vi "Min & Max Data display in graph.vi"() -> ()   [LabVIEW 2015]
panel:
  out "Waveform Graph":i32[](graph)
  # "Min & Max Data display in graph"
  # "Pardeep Kumar"
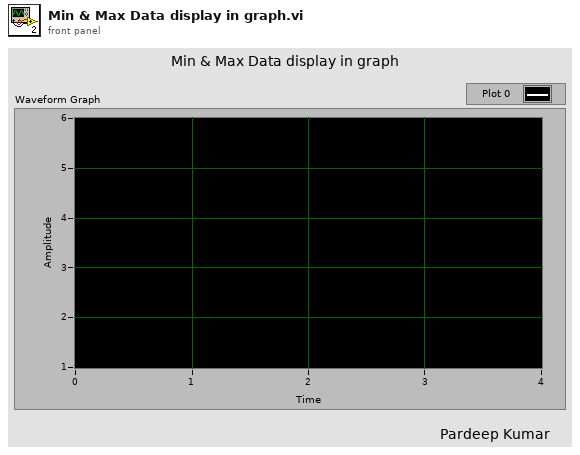
[diagram p1: front panel]
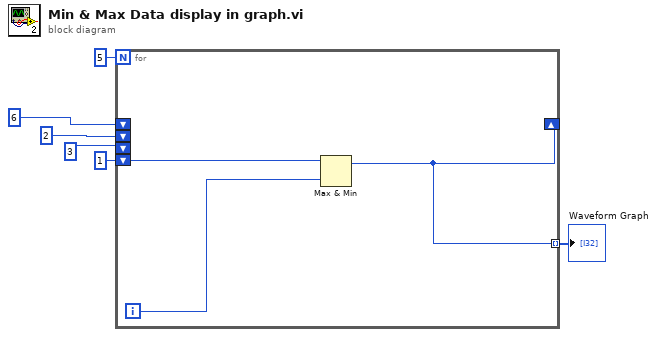
[diagram p0: block diagram]
diagram:
  n1 = for {
    N: 5 -> [_]
    shift-right: [w7] -> _
    shift-left: 1 -> [w8]
    shift-left: 3 -> [_]
    shift-left: 2 -> [_]
    shift-left: 6 -> [_]
    tunnel: [w7] -> w1 mode=indexing
    i -> [w9]
    n2 = Max & Min(x=w8, y=w9) -> (max(x,y)=w7:i32)  [unwired: 1 out]
  }
  "Waveform Graph" <- w1
